vi "Timeout Every 6 seconds.vi"() -> ()   [LabVIEW 2024]
panel:
  out "STOPPED?":bool
  in  "Stop Button":bool
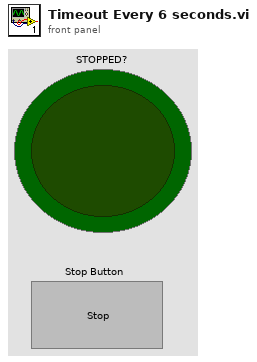
[diagram p1: front panel]
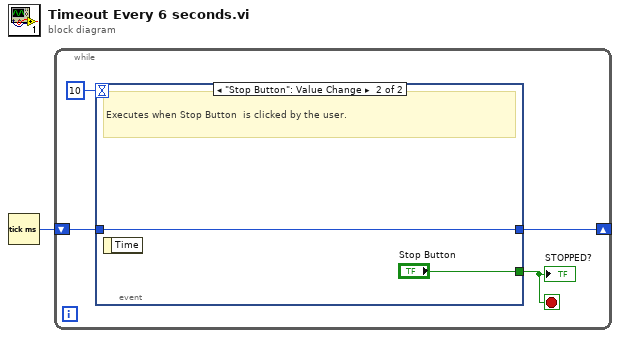
[diagram p0: block diagram]
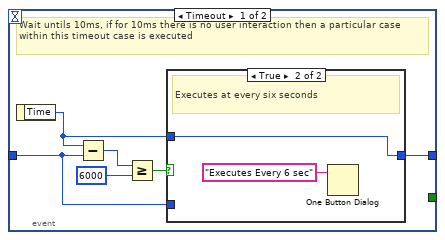
[diagram p2: hidden frame]
diagram:
  n1 = Tick Count (ms)() -> (millisecond timer value=w1:u32)
  n2 = while {
    shift-right: [w2] -> _
    shift-left: w1 -> [w3]
    stop <- w4 stop-if-true
    n3 = event shown="[1] \"Stop Button\": Value Change" {
      selector: _ -> [_ _]
      dyn-events: _ -> [_ _]
      timeout: 10 -> [_ _]
      tunnel: [_ "Stop Button"] -> w4
      tunnel: w3 -> [w6 w16]
      tunnel: [w7 w16] -> w2
      event Timeout {
        # "Wait untils 10ms, if for 10ms there is no user interaction then a particular case within this timeout case is executed"
        n4 = event-data() -> ("Time"=w8:u32)  [unwired: 1 in]
        n5 = Subtract(x=w8, y=w6) -> (x-y=w11:u32)
        n6 = Greater Or Equal?(x=w11, y=u32 6000) -> (x >= y?=w9:bool)
        n7 = case shown="True" w9 {
          tunnel: [w12 w14] -> w7
          tunnel: w8 -> [_ w14]
          tunnel: w6 -> [w12 _]
          frame False {
            # "Executes until timer condition encounters it as 6 seconds."
          }
          frame True {
            # "Executes at every six seconds"
            n8 = One Button Dialog(message="Executes Every 6 sec") -> ()  [unwired: 1 in, 1 out]
          }
        }
      }
      event "Stop Button": Value Change {
        # "Executes when Stop Button  is clicked by the user."
        n9 = event-data() -> ()  [unwired: 1 in, 1 out]
      }
    }
    "STOPPED?" <- w4
  }
